vi "Init_DAQ.vi"(8 "error in":errorcluster caption="entrée d'erreur") -> (0 "error out":errorcluster caption="sortie d'erreur")   [LabVIEW 2026]
uses:
  Controls/TypeDef_FGV.ctl
  <vilib>/DAQmx/create/channels.llb/DAQmx Create Channel (CO-Pulse Generation-Time).vi
  <vilib>/DAQmx/configure/timing.llb/DAQmx Timing (Implicit).vi
  FGV/FGV_DAQ_CO_Task.vi
  <vilib>/DAQmx/create/channels.llb/DAQmx Create Channel (DI-Digital Input).vi
  <vilib>/DAQmx/configure/timing.llb/DAQmx Timing (Change Detection).vi
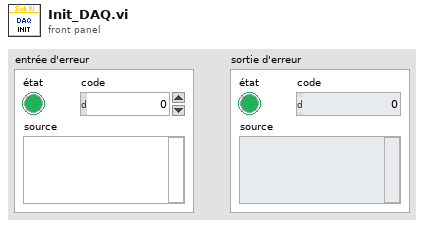
[diagram p1: front panel]
types:
  T1 = typedef "TypeDef_FGV.ctl" = enum16{"Initialize", "Write", "Read"}
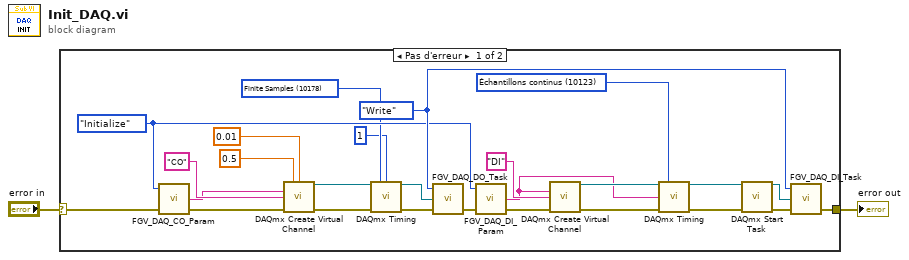
[diagram p0: block diagram]
diagram:
  n1 = case shown="Pas d'erreur" "error in" {
    selector: "error in" -> [w11 w29]
    tunnel: [w24 w29] -> w1
    frame No Error {
      w4 = 10178 items=["Finite Samples"=10178, "Continuous Samples"=10123, "Hardware Timed Single Point"=12522] ("sample mode")
      w20 = 10123 items=["Échantillons finis"=10178, "Échantillons continus"=10123, "Point par point avec cadencement matériel"=12522] ("sample mode")
      w12 = TypeDef_FGV."Initialize" ("Action")
      w25 = TypeDef_FGV."Write" ("Action")
      n2 = call "FGV_DAQ_CO_Param.vi"("error in"=w11, "Action"=w12) -> ("error out"=w10:errorcluster, "CO line"=w9:tag)  [unwired: 2 in]
      n3 = call-poly <vilib>:"DAQmx Create Virtual Channel.vi"("high time"=0.5, "low time"=0.01, "counter"=w9, "name to assign"="CO", "error in"=w10) -> ("task out"=w7:refnum<k21>, "error out"=w8:errorcluster)  [unwired: 9 in]
      n4 = call-poly <vilib>:"DAQmx Timing.vi"("task/channels in"=w7, "sample mode"=w4, "samples per channel"=1, "error in"=w8) -> ("task out"=w6:refnum<k21>, "error out"=w5:errorcluster)  [unwired: 10 in]
      n5 = call "FGV_DAQ_DO_Task.vi"("error in"=w5, "CO task"=w6, "Action"=w25) -> ("error out"=w27:errorcluster)  [unwired: 1 in, 1 out]
      n6 = call "FGV_DAQ_DI_Param.vi"("error in"=w27, "Action"=w12) -> ("error out"=w26:errorcluster, "DI line"=w15:tag)  [unwired: 2 in]
      n7 = call-poly <vilib>:"DAQmx Create Virtual Channel.vi"("lines"=w15, "name to assign"="DI", "error in"=w26) -> ("task out"=w22:refnum<k21>, "error out"=w21:errorcluster)  [unwired: 11 in]
      n8 = call-poly <vilib>:"DAQmx Timing.vi"("task/channels in"=w22, "sample mode"=w20, "rising edge physical channels"=w15, "error in"=w21) -> ("task out"=w19:refnum<k21>, "error out"=w18:errorcluster)  [unwired: 10 in]
      n9 = call <vilib>:"DAQmx Start Task.vi"("task/channels in"=w19, "error in"=w18) -> ("task out"=w17:refnum<k21>, "error out"=w16:errorcluster)  [unwired: 12 in]
      n10 = call "FGV_DAQ_DI_Task.vi"("error in"=w16, "DI task"=w17, "Action"=w25) -> ("error out"=w24:errorcluster)  [unwired: 1 in, 1 out]
    }
    frame Error {
    }
  }
  "error out" <- w1
